vi "Make_Box_Visible.vi"(1 "mm Per Pixel":dbl format="%.2f", 2 "X":cluster{"Max":dbl, "Min":dbl}) -> (0 "Array":dbl[](array[numeric]))   [LabVIEW 2010]
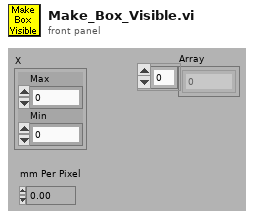
[diagram p1: front panel]
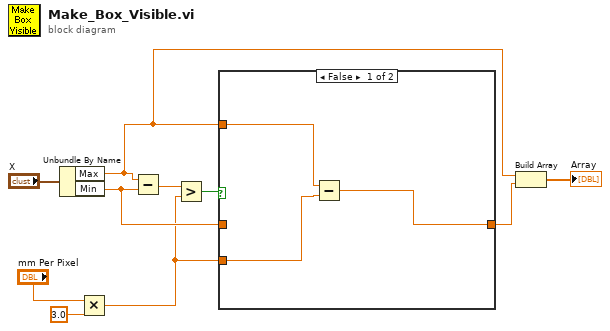
[diagram p0: block diagram]
diagram:
  n1 = Unbundle By Name("X") -> ("Max"=w2:dbl, "Min"=w5:dbl)
  n2 = Multiply(x="mm Per Pixel", y=3.0) -> (x*y=w3:dbl)
  n3 = Subtract(x=w2, y=w5) -> (x-y=w7:dbl)
  n4 = Greater?(x=w7, y=w3) -> (0:w6:bool)
  n5 = case shown="False" w6 {
    tunnel: w2 -> [w13 _]
    tunnel: w5 -> [_ w14]
    tunnel: [w11 w14] -> w4
    tunnel: w3 -> [w12 _]
    frame False {
      n6 = Subtract(x=w13, y=w12) -> (x-y=w11:dbl)
    }
    frame True {
    }
  }
  n7 = Build Array(w2, w4) -> (→"Array":dbl[])
